vi "MAIN_static_friction.vi"() -> ()   [LabVIEW 2019]
uses:
  <vilib>/myRIO/Instrument Drivers/Onboard IO/AO/AO.lvlib
  <vilib>/myRIO/Instrument Drivers/Onboard IO/Encoder/Encoder.lvlib
  <vilib>/myRIO/Instrument Drivers/Onboard IO/AI/AI.lvlib
  <vilib>/addons/control/pid/NI_PID_pid.lvlib
  <vilib>/Analysis/3filter.llb/Filter Passband Type.ctl
  <vilib>/Analysis/NI_AALBase.lvlib
  <vilib>/ptbypt/NI_PtbyPt.lvlib
  <vilib>/platform/TimedLoop/XDataNode/XDataNode.xnode
  <vilib>/Platform/TimedLoop/XDataNode/timing_clust.ctl
  <vilib>/Platform/TimedLoop/XDataNode/XDNodeRunTimeDep.lvlib
  <vilib>/Platform/TimedLoop/XDataNode/wakeup.ctl
  <vilib>/Platform/TimedLoop/XDataNode/nitl_modes.ctl
  <vilib>/myRIO/Common/Instrument Driver Framework/myRIO v1.0/Encoder/typedefs/Encoder Signal Mode.ctl
  <vilib>/myRIO/Instrument Drivers/Onboard IO/AO/vis/myRIO AO Open.xnode
  <vilib>/myRIO/Instrument Drivers/Onboard IO/AO/typedefs/AO Reference.ctl
  <vilib>/myRIO/Common/Instrument Driver Framework/Utilities/typedefs/Analog Scaling Constants List.ctl
  <vilib>/myRIO/Common/Instrument Driver Framework/Utilities/typedefs/Analog Scaling Constants.ctl
  <vilib>/myRIO/Common/Instrument Driver Framework/myRIO v1.0/AO/typedefs/AO Channels List.ctl
  <vilib>/myRIO/Common/Instrument Driver Framework/myRIO v1.0/AO/typedefs/AO Channels Enum.ctl
  <vilib>/myRIO/Common/Instrument Driver Framework/Utilities/typedefs/myRIO Generic Hardware Reference.ctl
  <vilib>/myRIO/Common/Instrument Driver Framework/Utilities/typedefs/myRIO v1.0 Reference.ctl
  <vilib>/myRIO/Common/Instrument Driver Framework/Utilities/typedefs/Generic FPGA Reference.ctl
  <vilib>/myRIO/Common/Instrument Driver Framework/Utilities/typedefs/Hardware Version Enum.ctl
  <vilib>/userDefined/High Color/nirio_resource_hc.ctl
  <vilib>/myRIO/Common/Instrument Driver Framework/myRIO v1.0/AO/vis/myRIO v1.1 Open AO.vi
  <vilib>/myRIO/Instrument Drivers/Onboard IO/AI/vis/myRIO AI Open.xnode
  <vilib>/myRIO/Instrument Drivers/Onboard IO/AI/typedefs/AI Reference.ctl
  <vilib>/myRIO/Common/Instrument Driver Framework/myRIO v1.0/AI/typedefs/AI Channels List.ctl
  <vilib>/myRIO/Common/Instrument Driver Framework/myRIO v1.0/AI/typedefs/AI Channels Enum.ctl
  <vilib>/myRIO/Common/Instrument Driver Framework/myRIO v1.0/AI/vis/myRIO v1.1 Open AI.vi
  Shared VIs/TypeDef_TDMS_States.ctl
  TypeDef_Actions.ctl
  Shared VIs/ENPID/PID_Settings.ctl
  Shared VIs/ENPID/OutputRange.ctl
  Shared VIs/ENPID/VelocityEstimate.ctl
  Shared VIs/ENPID/DPartVariable.ctl
  Shared VIs/ENPID/NonLinearGain.ctl
  Shared VIs/ENPID/NonLinearGainParams.ctl
  Shared VIs/ENPID/Gains.ctl
  TypeDef_Current-Direction.ctl
panel:
  in  "Pos Difference \nThreshold [deg]":dbl=1.0 min=0.0 max=1.0 step=0.01 format="%#_13g"
  in  "Actions":T1
  in  "Current Direction":T2
  out "Position End [deg] Chart":dbl(graph)
  out "Position End [deg]":dbl
  out "Initial Position [deg]":dbl
  out "Velocity [deg/s] Chart":dbl(graph)
  in  "Stop saving data":bool
  in  "Save data?":bool
  in  "File Storage Name":string
  out "Final Current Setpoint":dbl
  out "Boolean: Apply Current":bool
  out "Boolean: Move":bool
  out "Position Difference [deg]":dbl
  in  "move":bool
  out "Profile Complete?":bool
  out "Velocity [deg/s]":dbl
  out "Current Setpoint [A]":dbl
  out "Position [deg] Chart":dbl(graph)
  out "Current [A] Chart":dbl(graph)
  out "Position [deg]":dbl
  in  "stop":bool
  out "Current [A]":dbl
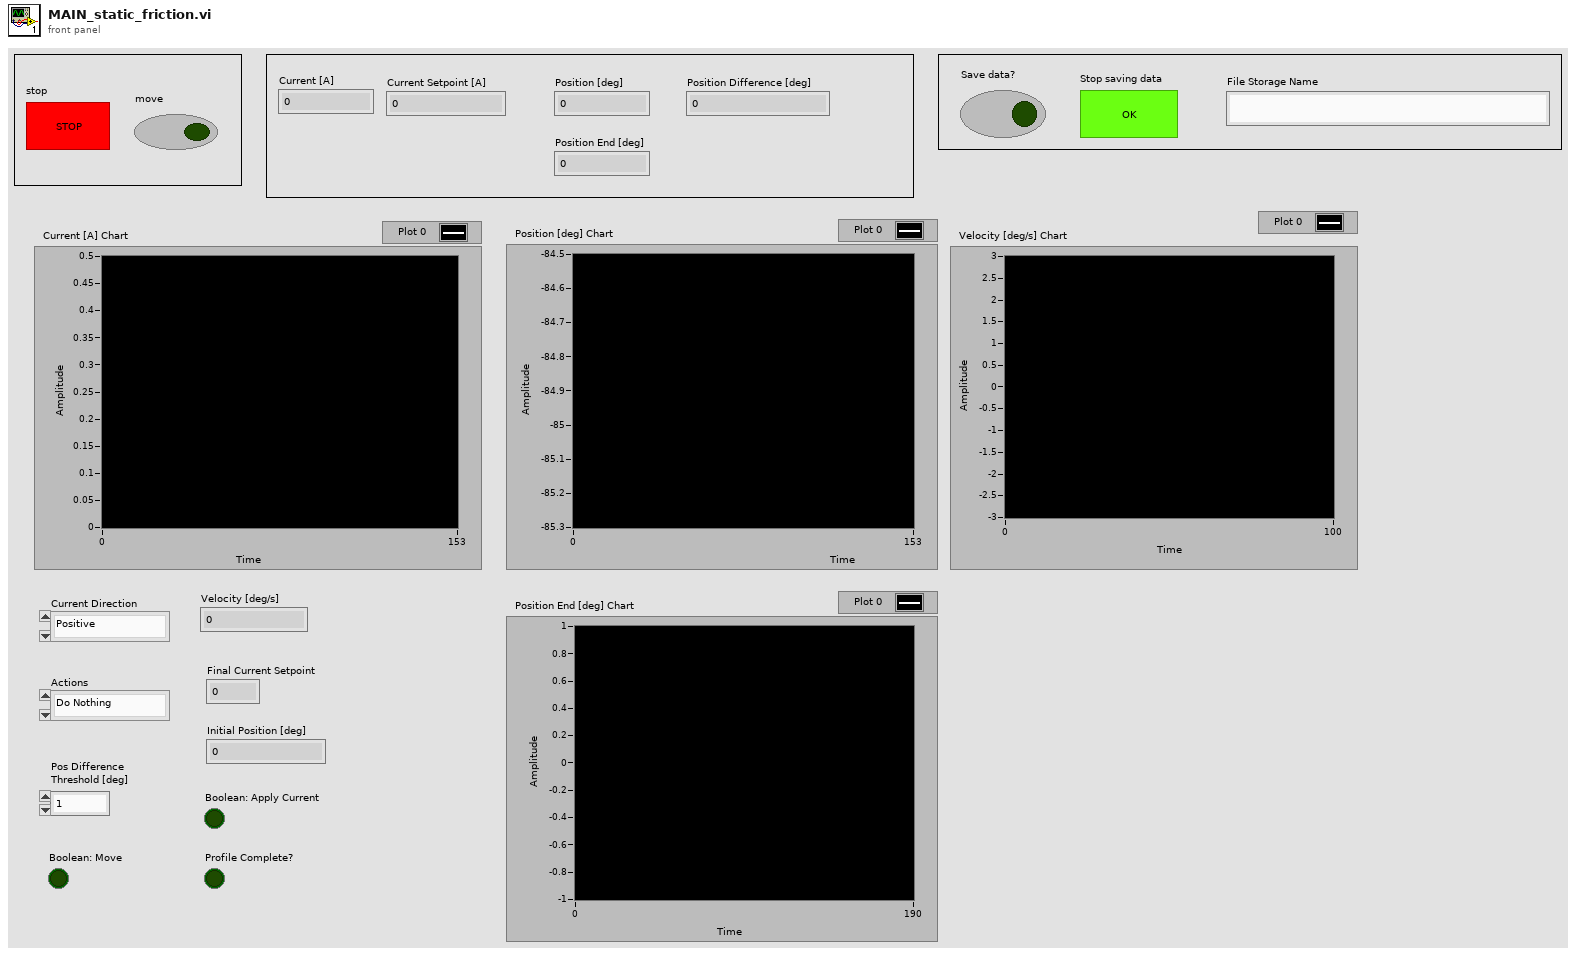
[diagram p1: front panel]
types:
  T1 = typedef "TypeDef_Actions.ctl" = enum16{"Do Nothing", "Move", "Wait", "Apply Current"}
  T2 = typedef "TypeDef_Current-Direction.ctl" = enum16{"Positive", "Negative"}
  T3 = typedef "nirio_resource_hc.ctl" = tag
  T4 = typedef "Hardware Version Enum.ctl" = enum16{"Unknown", "myRIO-1900", "myRIO-1950", "roboRIO", "NI ELVIS RIO CM", "ELVIS III"}
  T5 = typedef "TypeDef_TDMS_States.ctl" = enum16{"WaitingForCreate", "Create", "Buffering", "Flushing", "Write", "Close"}
  T6 = enum16{"open", "open or create", "create or replace", "create", "open (read-only)"}
  T7 = typedef "XDNodeRunTimeDep.lvlib/timing_clust.ctl" = cluster{"Expected End [f-1]":u64, "Actual End [f-1]":u64, "Finished Late? [f-1]":bool, "Expected End [i-1]":u64, "Actual End [i-1]":u64, "Finished Late? [i-1]":bool, "Expected Start [i]":u64, "Actual Start [i]":u64, "Expected Start [f]":u64, "Actual Start [f]":u64, "Source Name":string, "Structure Name":string, "Period":i64, "Deadline":i64, "Offset":i64, "Start":i64, "Priority":i32, "Timeout":i32, "Mode":T8, "Wakeup Reason":T9, "Error":errorcluster, "Source Type":string, "Secondary Source Type":string, "Global End Time":u64, "Global Start Time":u64, "Frame Duration":u64, "Iteration Duration":u64, "Assigned CPU":i32, "I/O Scan Engine Mode":u32}
  T8 = typedef "XDNodeRunTimeDep.lvlib/nitl_modes.ctl" = enum32{"No Change", "Process missed periods, maintain original phase", "Discard missed periods, maintain original phase", "Process missed periods, ignore original phase", "Discard missed periods, ignore original phase"}
  T9 = typedef "XDNodeRunTimeDep.lvlib/wakeup.ctl" = enum32{"Normal", "Aborted", "Asynchronous wakeup", "Timing source error", "Timed loop error", "Timeout"}
  T10 = typedef "NI_AALBase.lvlib/Filter Passband Type.ctl" = enum32{"Lowpass", "Highpass", "Bandpass", "Bandstop"}
  T11 = typedef "PID_Settings.ctl" = cluster{"Gains":T12, "Non-linear gain":T13, "D-Part variable":T15, "Velocity estimate dy/dt":T16, "Anti reset windup":bool, "I-Part error band":dbl, "Output range":T17}
  T12 = typedef "Gains.ctl" = cluster{"K(e)":dbl, "Kp":dbl, "Ki":dbl, "Kd":dbl}
  T13 = typedef "NonLinearGainParams.ctl" = cluster{"Non-linear gain P":T14, "Non-linear gain I":T14, "Non-linear gain D":T14}
  T14 = typedef "NonLinearGain.ctl" = enum16{"exponential", "quadratic", "off"}
  T15 = typedef "DPartVariable.ctl" = enum16{"error", "process variable"}
  T16 = typedef "VelocityEstimate.ctl" = enum16{"derivative", "external"}
  T17 = typedef "OutputRange.ctl" = cluster{"output high":dbl, "output low":dbl}
  T18 = typedef "Encoder Signal Mode.ctl" = enum16{"Quadrature phase signal", "Step and direction signal"}
  T19 = typedef "AO.lvlib/AO Reference.ctl" = cluster{"myRIO Reference":T20, "AO Channel List":T23, "AO Scaling Constant List":T25}
  T20 = typedef "myRIO Generic Hardware Reference.ctl" = cluster{"myRIO Model":T4, "myRIO Hardware Reference":T21}
  T21 = typedef "myRIO v1.0 Reference.ctl" = cluster{"Generic FPGA Reference":T22, "Allow multiple opens":bool}
  T22 = typedef "Generic FPGA Reference.ctl" = refnum<k20>
  T23 = typedef "AO Channels List.ctl" = T24[]
  T24 = typedef "AO Channels Enum.ctl" = enum16{"Not Connected", "AudioOut/Left", "AudioOut/Right", "C/AO0", "C/AO1", "A/AO0", "A/AO1", "B/AO0", "B/AO1"}
  T25 = typedef "Analog Scaling Constants List.ctl" = T26[]
  T26 = typedef "Analog Scaling Constants.ctl" = cluster{"LSB Weight (Volts)":dbl, "Offset (Volts)":dbl, "Signed?":bool}
  T27 = typedef "Encoder.lvlib/Encoder Reference.ctl" = cluster{"myRIO Reference":T20, "Encoder Channels Enum":T28}
  T28 = typedef "Encoder Channels Enum.ctl" = enum16{"Not Connected", "C/ENC0", "C/ENC1", "A/ENC", "A/ENC0", "A/ENC1", "A/ENC2", "A/ENC3", "A/ENC4", "A/ENC5", "A/ENC6", "A/ENC7", "A/ENC8", "A/ENC9", "B/ENC", "B/ENC0", "B/ENC1", "B/ENC2", "B/ENC3", "B/ENC4", "B/ENC5", "B/ENC6", "B/ENC7", "B/ENC8", "B/ENC9", "DIO/ENC0", "DIO/ENC1", "DIO/ENC2", "DIO/ENC3", "DIO/ENC4"}
  T29 = typedef "AI.lvlib/AI Reference.ctl" = cluster{"myRIO Reference":T20, "AI Channels List":T30, "AI Scaling Constants List":T25}
  T30 = typedef "AI Channels List.ctl" = T31[]
  T31 = typedef "AI Channels Enum.ctl" = enum16{"Not Connected", "AudioIn/Left", "AudioIn/Right", "C/AI0", "C/AI1", "A/AI0", "A/AI1", "A/AI2", "A/AI3", "A/AI4", "A/AI5", "A/AI6", "A/AI7", "B/AI0", "B/AI1", "B/AI2", "B/AI3", "B/AI4", "B/AI5", "B/AI6", "B/AI7", "AI/AI0", "AI/AI1", "AI/AI2", "AI/AI3", "A/AI0 (DIFF)", "A/AI1 (DIFF)", "A/AI2 (DIFF)", "A/AI3 (DIFF)", "B/AI0 (DIFF)", "B/AI1 (DIFF)", "B/AI2 (DIFF)", "B/AI3 (DIFF)"}
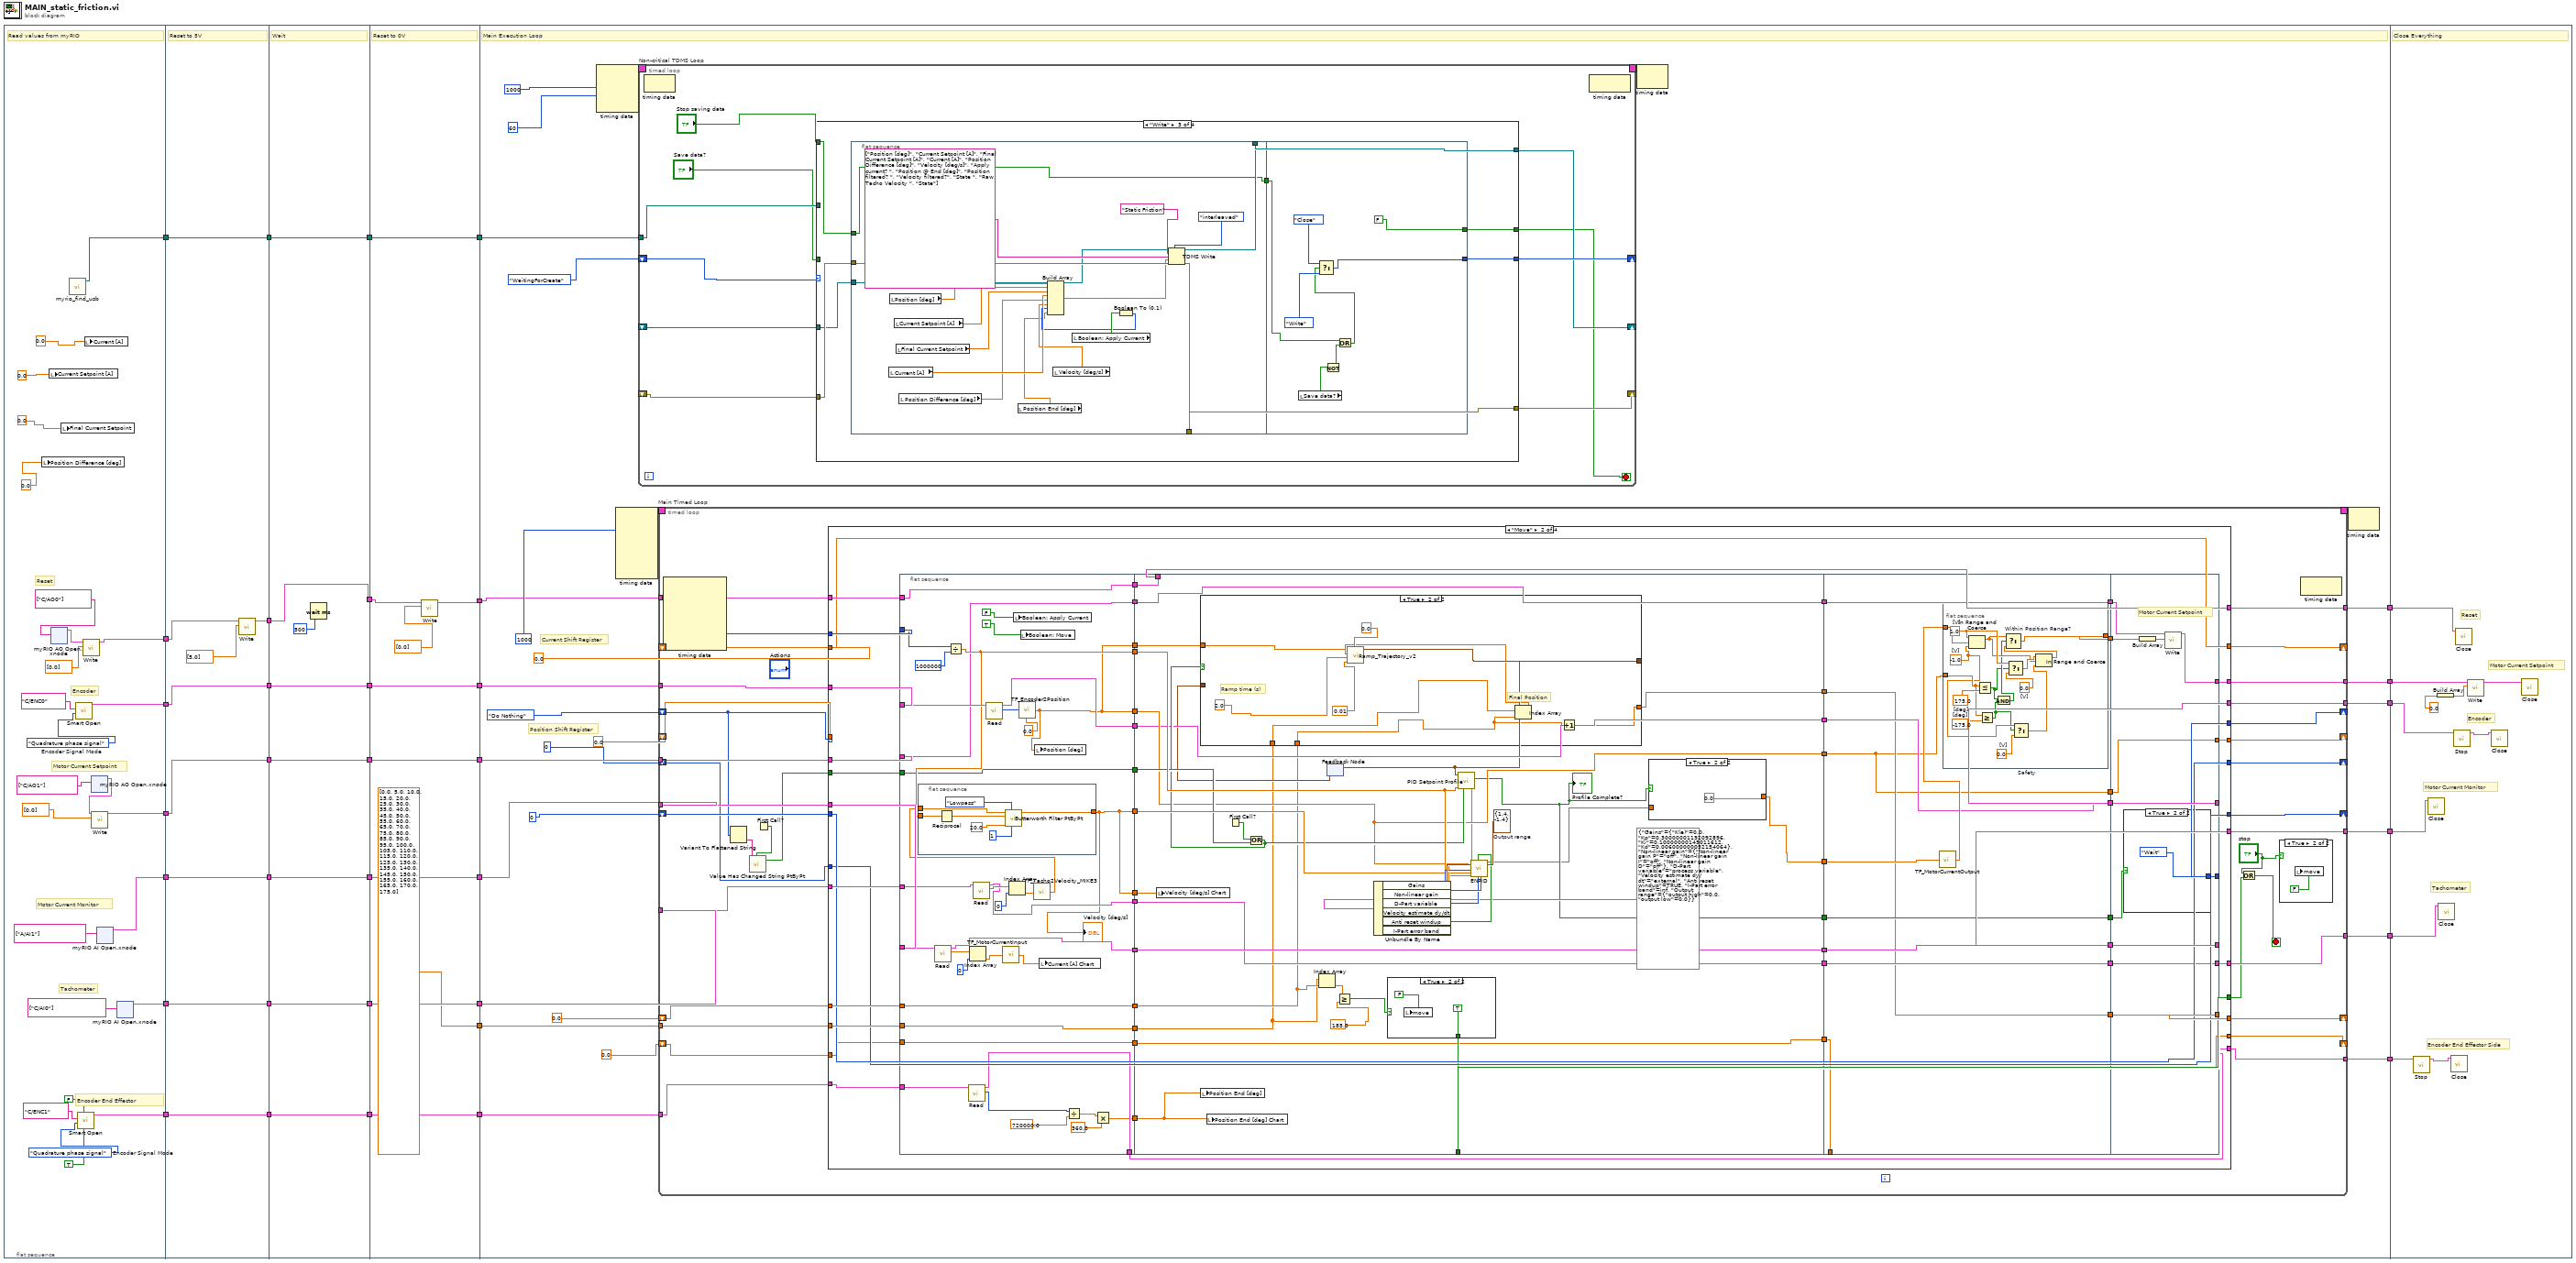
[diagram p0: block diagram]
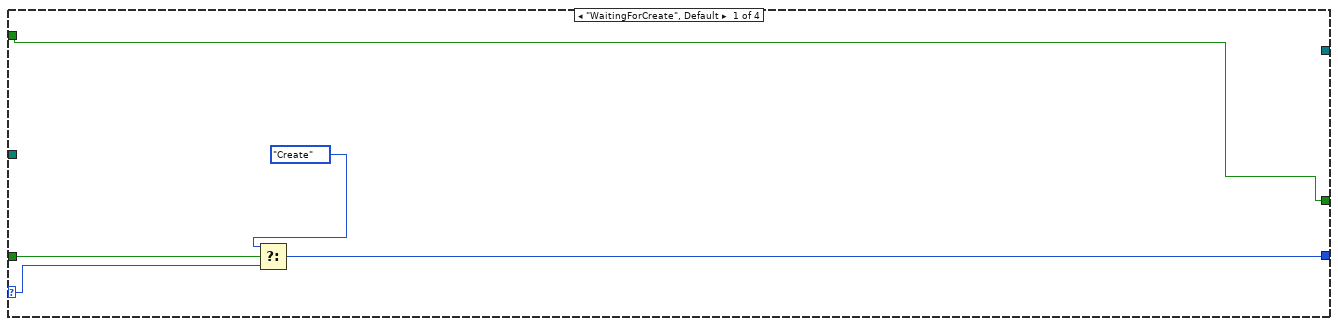
[diagram p2: hidden frame]
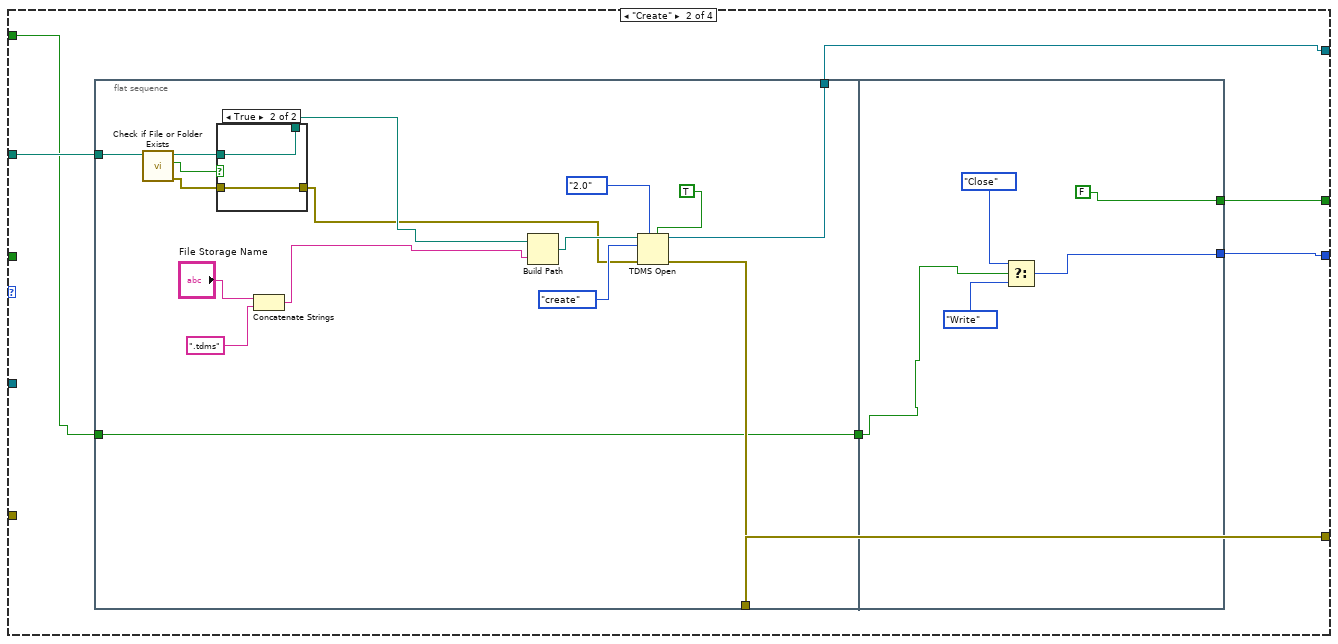
[diagram p3: hidden frame]
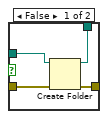
[diagram p4: hidden frame]
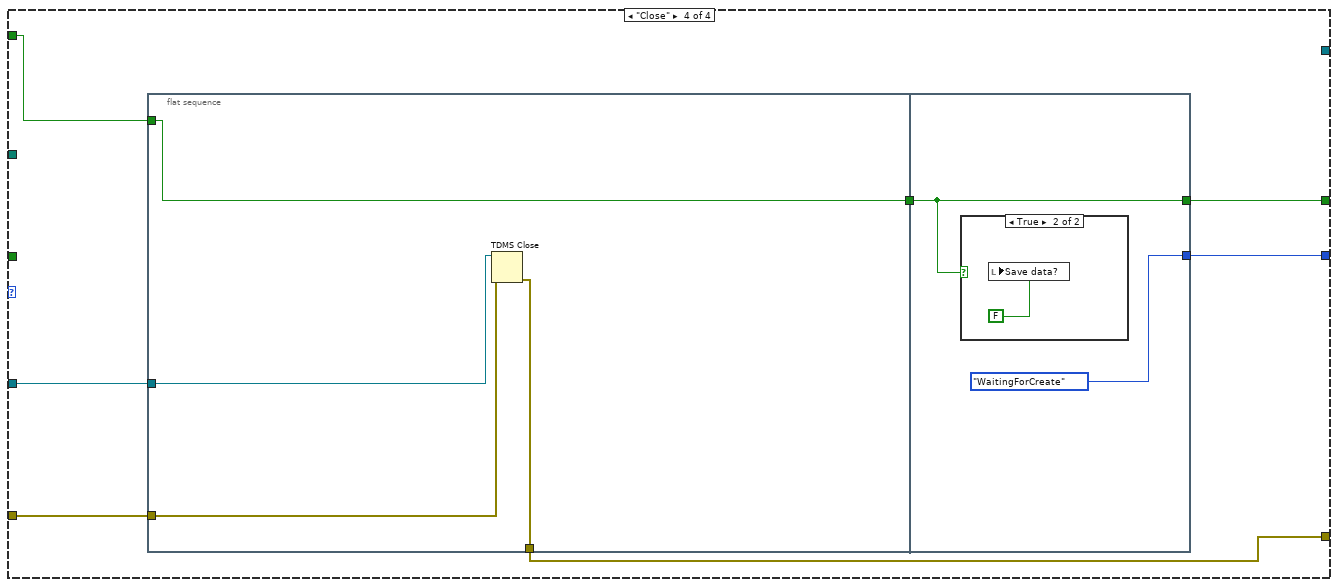
[diagram p5: hidden frame]
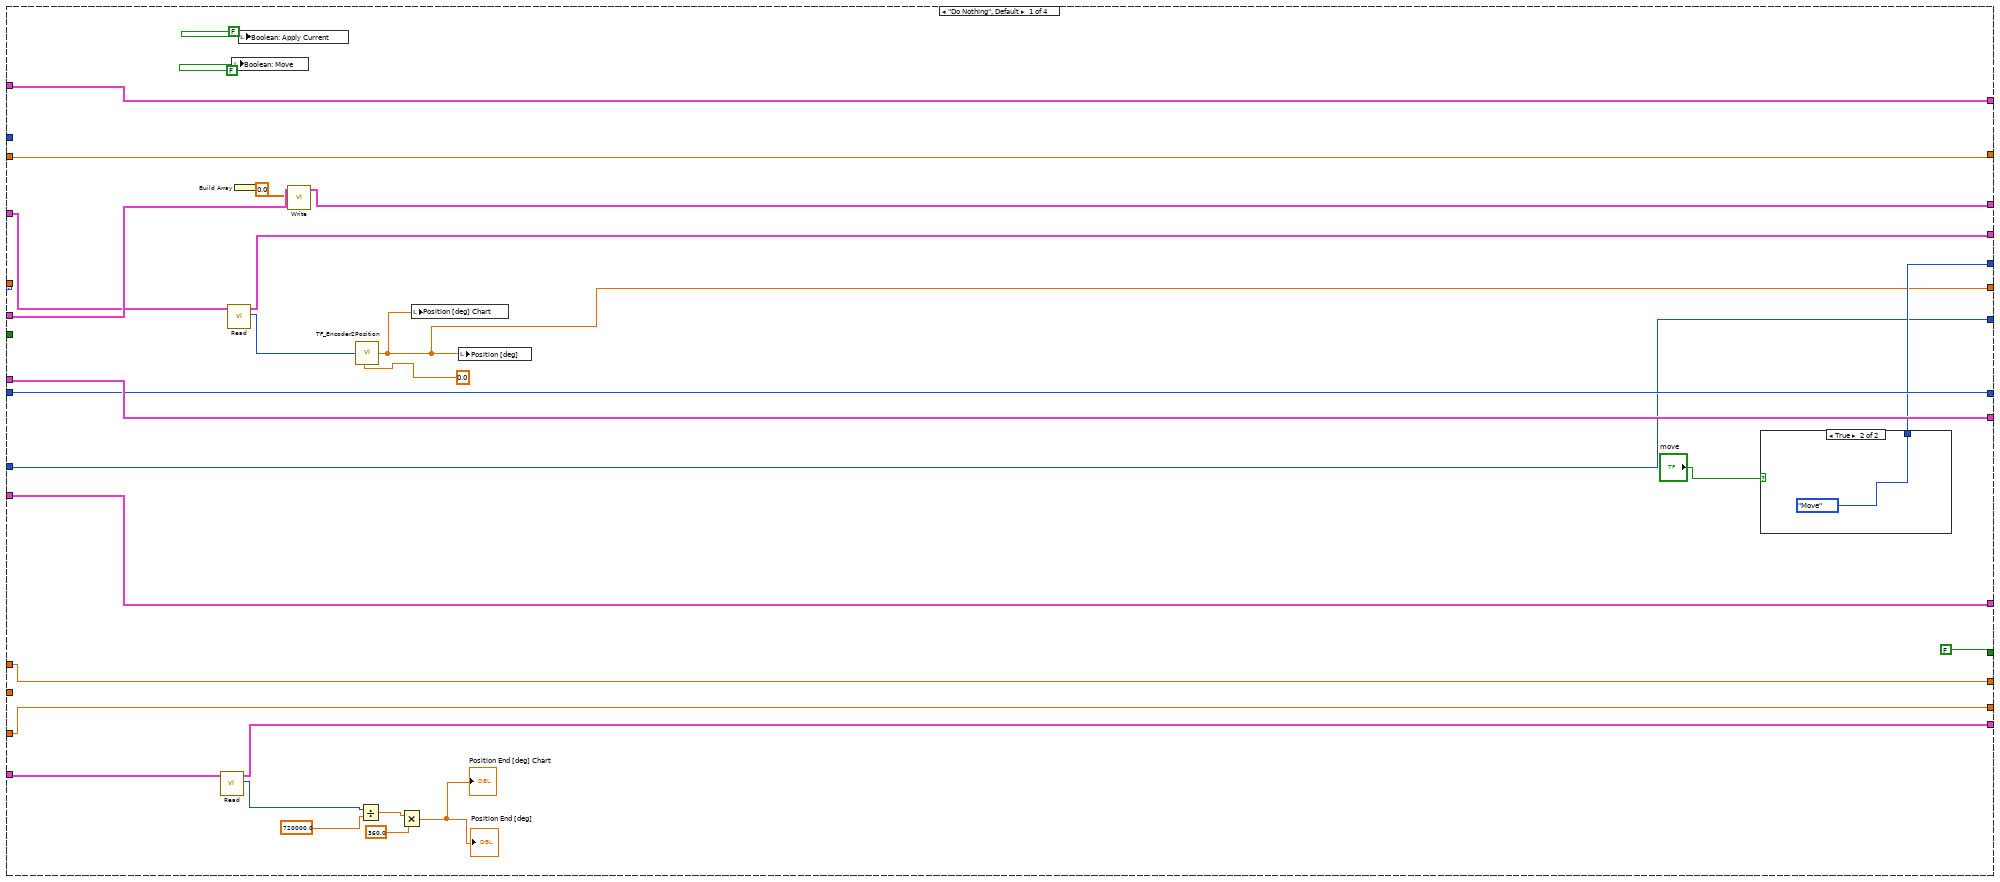
[diagram p8: hidden frame]
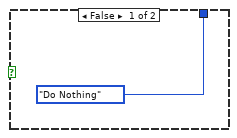
[diagram p9: hidden frame]
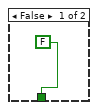
[diagram p10: hidden frame]
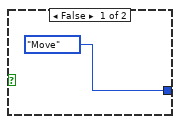
[diagram p13: hidden frame]
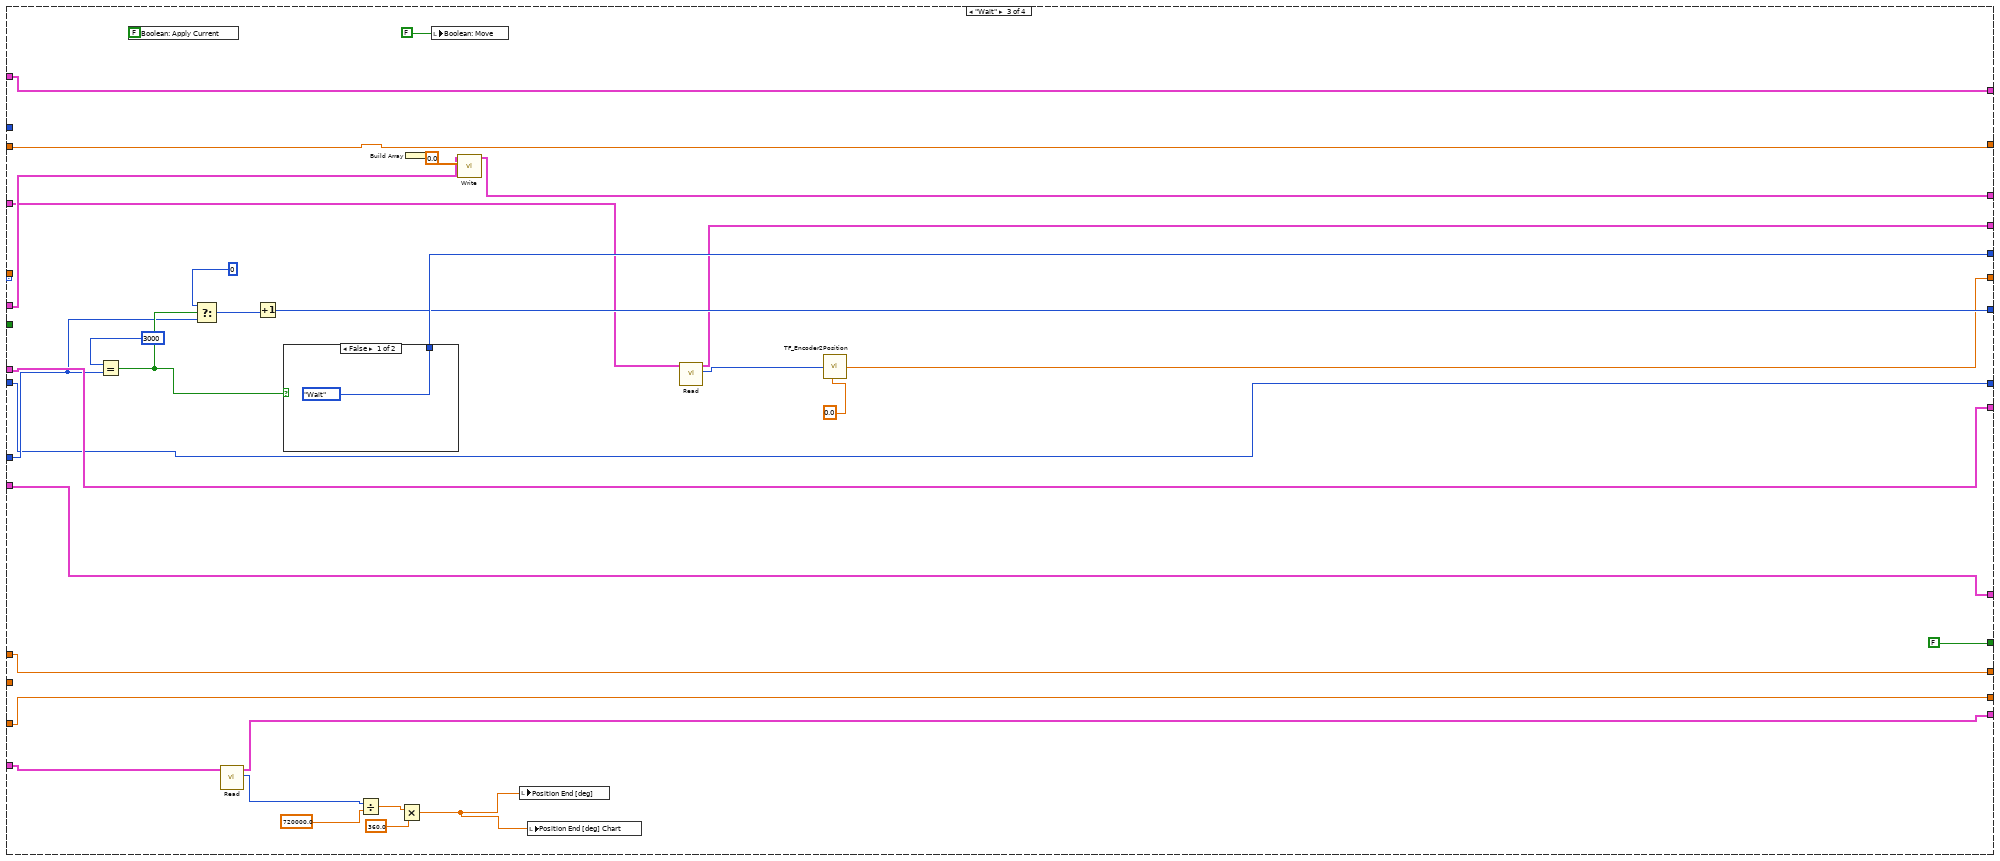
[diagram p14: hidden frame]
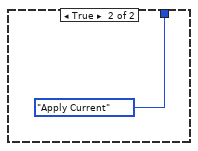
[diagram p15: hidden frame]
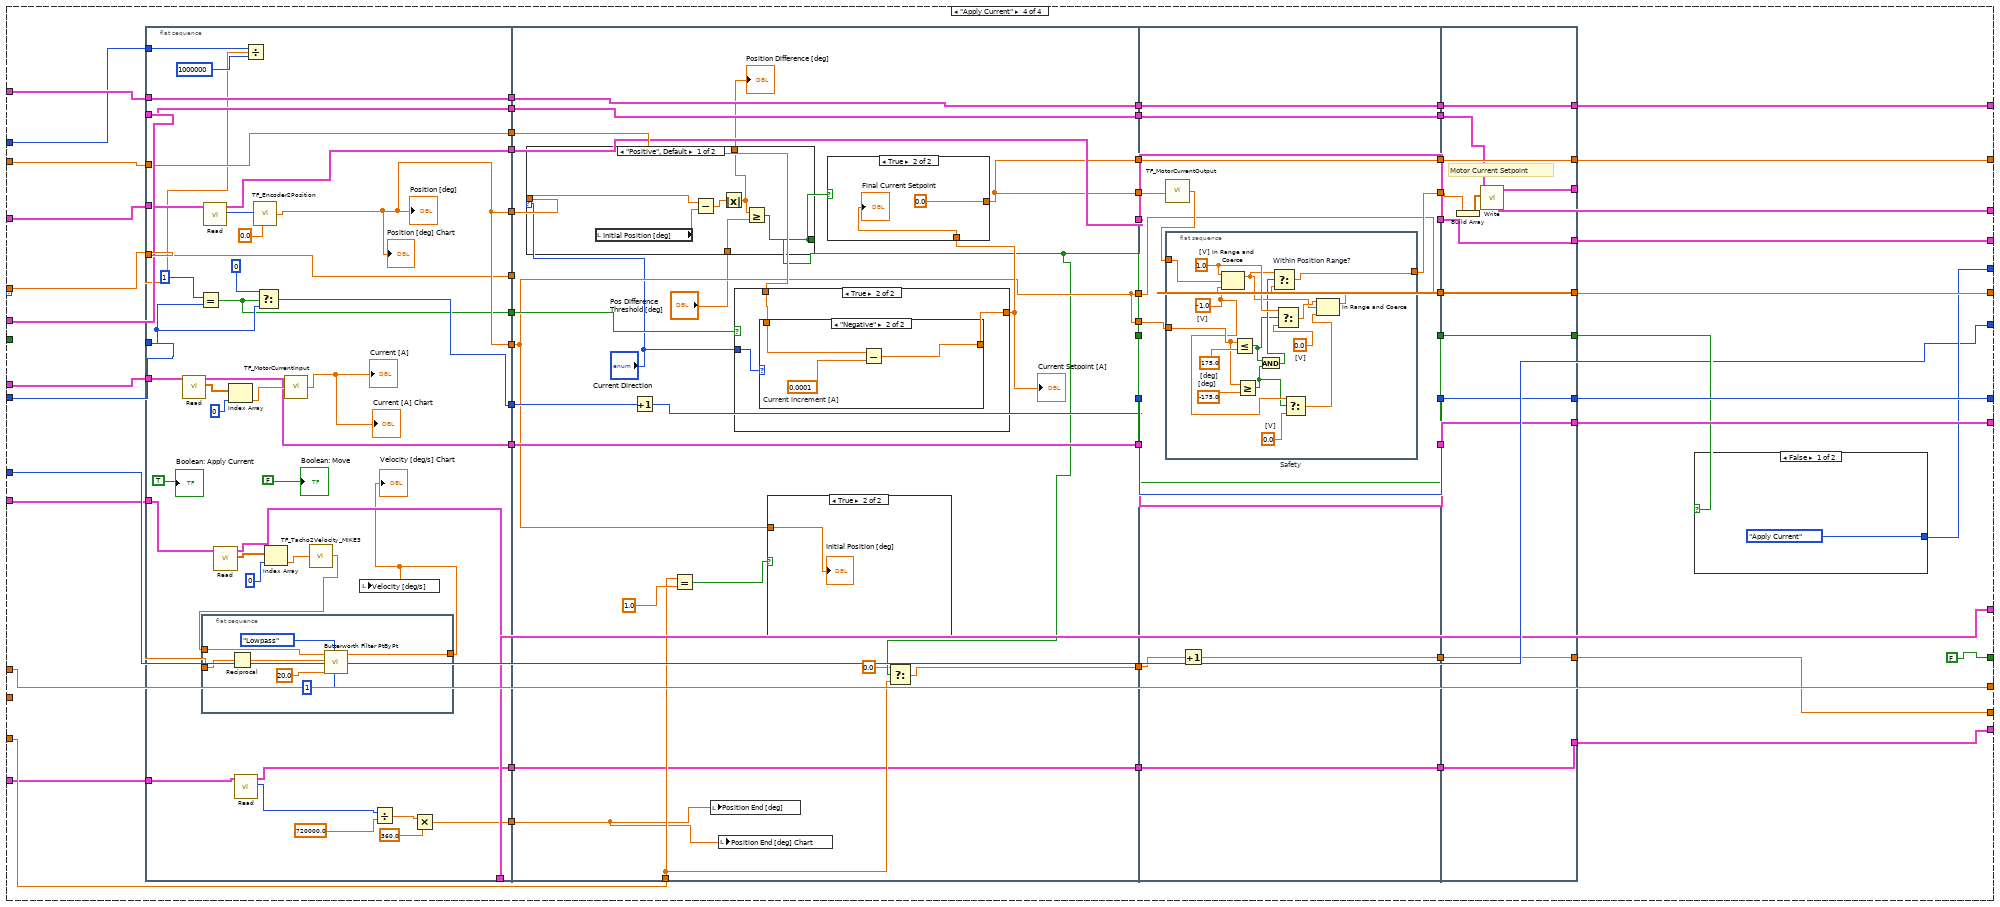
[diagram p16: hidden frame]
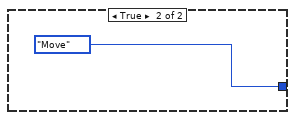
[diagram p17: hidden frame]
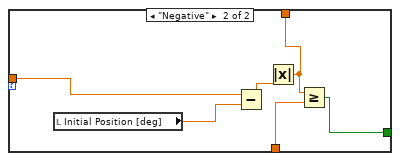
[diagram p19: hidden frame]
diagram:
  n1 = flat-sequence {
    tunnel: [w57] -> w35
    tunnel: [w54] -> w31
    tunnel: [w50] -> w30
    tunnel: [w48] -> w29
    tunnel: [w46] -> w12
    tunnel: [w45] -> w6
    tunnel: [w36] -> w2
    tunnel: w35 -> [w140]
    tunnel: [w139] -> w33
    tunnel: w31 -> [w138]
    tunnel: w30 -> [w137]
    tunnel: w29 -> [w136]
    tunnel: [w138] -> w26
    tunnel: [w137] -> w23
    tunnel: [w136] -> w20
    tunnel: [w135] -> w13
    tunnel: w12 -> [w135]
    tunnel: [w134] -> w7
    tunnel: w6 -> [w134]
    tunnel: [w133] -> w3
    tunnel: w2 -> [w133]
    tunnel: [w148] -> w34
    tunnel: w33 -> [w148]
    tunnel: [w147] -> w27
    tunnel: w26 -> [w147]
    tunnel: [w146] -> w24
    tunnel: w23 -> [w146]
    tunnel: [w145] -> w21
    tunnel: w20 -> [w145]
    tunnel: [w144] -> w14
    tunnel: w13 -> [w144]
    tunnel: [w143] -> w8
    tunnel: w7 -> [w143]
    tunnel: [w142] -> w4
    tunnel: w3 -> [w142]
    tunnel: w34 -> [w158]
    tunnel: [w157] -> w32
    tunnel: [w156] -> w28
    tunnel: w27 -> [w156]
    tunnel: [w155] -> w25
    tunnel: w24 -> [w155]
    tunnel: [w154] -> w22
    tunnel: w21 -> [w154]
    tunnel: [w153] -> w15
    tunnel: w14 -> [w153]
    tunnel: [dbl[] [0.0, 5.0, 10.0, 15.0, 20.0, 25.0, 30.0, 35.0, 40.0, 45.0, 50.0, 55.0, 60.0, 65.0, 70.0, 75.0, 80.0, 85.0, 90.0, 95.0, 100.0, 105.0, 110.0, 115.0, 120.0, 125.0, 130.0, 135.0, 140.0, 145.0, 150.0, 155.0, 160.0, 165.0, 170.0, 175.0]] -> w10
    tunnel: [w151] -> w9
    tunnel: w8 -> [w151]
    tunnel: [w150] -> w5
    tunnel: w4 -> [w150]
    tunnel: w32 -> [w181]
    tunnel: w28 -> [w185]
    tunnel: w25 -> [w184]
    tunnel: w22 -> [w175]
    tunnel: [w180] -> w19
    tunnel: [w179] -> w18
    tunnel: [w178] -> w17
    tunnel: [w177] -> w16
    tunnel: w15 -> [w176]
    tunnel: [w174] -> w11
    tunnel: w10 -> [w173]
    tunnel: w9 -> [w166]
    tunnel: w5 -> [w162]
    tunnel: [w161] -> w1
    tunnel: w19 -> [w805]
    tunnel: w18 -> [w800]
    tunnel: w17 -> [w799]
    tunnel: w16 -> [w798]
    tunnel: w11 -> [w797]
    tunnel: w1 -> [w795]
    frame #0 {
      w39 = Encoder_Signal_Mode."Quadrature phase signal"  # Encoder Signal Mode
      w55 = Encoder_Signal_Mode."Quadrature phase signal"  # Encoder Signal Mode
      # "Encoder End Effector"
      # "Tachometer"
      # "Motor Current Monitor"
      # "Motor Current Setpoint"
      # "Encoder"
      # "Reset"
      # "Read values from myRIO"
      n2 = local write "Position Difference [deg]"(0.0) -> ()
      n3 = local write "Current Setpoint [A]"(0.0) -> ()
      n4 = xnode "myRIO AO Open.xnode"("Channel Names"=tag[] ["C/AO0"]) -> ("AO Ref Out"=w59:T19)  [unwired: 2 in, 1 out]
      n5 = local write "Final Current Setpoint"(0.0) -> ()
      n6 = call "myrio_find_usb.vi"() -> ("Largest USB Partition Path"=w45:path)  [unwired: 9 in, 2 out]
      n7 = call <vilib>:"Smart Open.vi"("Encoder Signal Mode"=w55, "Channel Name"=tag "C/ENC0") -> ("Encoder Ref Out"=w54:T27)  [unwired: 8 in, 1 out]
      n8 = call <vilib>:"Smart Open.vi"("Start Counter"=TRUE, "Allow multiple opens?"=FALSE, "Encoder Signal Mode"=w39, "Channel Name"=tag "C/ENC1") -> ("Encoder Ref Out"=w36:T27)  [unwired: 6 in, 1 out]
      n9 = call <vilib>:"Write.vi"("Values"=dbl[] [0.0], "AO Ref In"=w59) -> ("AO Ref Out"=w57:T19)  [unwired: 7 in, 1 out]
      n10 = local write "Current [A]"(0.0) -> ()
      n11 = xnode "myRIO AO Open.xnode"("Channel Names"=tag[] ["C/AO1"]) -> ("AO Ref Out"=w52:T19)  [unwired: 2 in, 1 out]
      n12 = call <vilib>:"Write.vi"("Values"=dbl[] [0.0], "AO Ref In"=w52) -> ("AO Ref Out"=w50:T19)  [unwired: 7 in, 1 out]
      n13 = xnode "myRIO AI Open.xnode"("Channel Names"=tag[] ["A/AI1"]) -> ("AI Ref Out"=w48:T29)  [unwired: 2 in, 1 out]
      n14 = xnode "myRIO AI Open.xnode"("Channel Names"=tag[] ["C/AI0"]) -> ("AI Ref Out"=w46:T29)  [unwired: 2 in, 1 out]
    }
    frame #1 {
      # "Reset to 5V"
      n15 = call <vilib>:"Write.vi"("Values"=dbl[] [5.0], "AO Ref In"=w140) -> ("AO Ref Out"=w139:T19)  [unwired: 7 in, 1 out]
    }
    frame #2 {
      # "Wait"
      n16 = Wait (ms)(milliseconds to wait=500) -> ()  [unwired: 1 out]
    }
    frame #3 {
      # "Reset to 0V"
      n17 = call <vilib>:"Write.vi"("Values"=dbl[] [0.0], "AO Ref In"=w158) -> ("AO Ref Out"=w157:T19)  [unwired: 7 in, 1 out]
    }
    frame #4 {
      # "Position Shift Register"
      # "Current Shift Register"
      # "Main Execution Loop"
      n18 = node-c288(1000, 60) -> (w170:T7)  [unwired: 2 in]
      n19 = node-c288(1000) -> (w188:T7)  [unwired: 6 in]
      n20 = timed-loop "Non-critical TDMS Loop" {
        timing: w170 -> [_]
        timing-out: [_] -> w169
        tunnel: w166 -> [w196]
        shift-right: [w198] -> _
        shift-left: TypeDef_TDMS_States."WaitingForCreate" ("TDMS States") -> [w197]
        shift-right: [w195] -> _
        shift-left: _ -> [w192]
        shift-right: [w194] -> _
        shift-left: _ -> [w193]
        stop <- w191 stop-if-true
        n21 = node-c288() -> ()  [unwired: 1 in, 1 out]
        n22 = case shown="\"Write\"" w197 {
          selector: w197 -> [w201 _ _ _]
          tunnel: "Save data?" -> [w202 _ _ _]
          tunnel: [w200 w207 w242 w275] -> w198
          tunnel: w196 -> [_ w210 _ _]
          tunnel: [_ w208 w243 _] -> w195
          tunnel: [_ w209 w245 w276] -> w194
          tunnel: w193 -> [_ _ w244 w277]
          tunnel: w192 -> [_ _ w240 w278]
          tunnel: [w199 w206 w241 w274] -> w191
          tunnel: "Stop saving data" -> [w199 w204 w238 w273]
          frame "WaitingForCreate", Default {
            n23 = Select(t=TypeDef_TDMS_States."Create" ("TDMS States"), s=w202, f=w201) -> (s? t:f=w200:T5)
          }
          frame "Create" {
            n24 = flat-sequence {
              tunnel: w210 -> [w226]
              tunnel: [w214] -> w209
              tunnel: [w213] -> w208
              tunnel: [w211] -> w205
              tunnel: w204 -> [w211]
              tunnel: [w235] -> w207
              tunnel: [FALSE] -> w206
              tunnel: w205 -> [w233]
              frame #0 {
                n25 = call <vilib>:"Check if File or Folder Exists.vi"("path"=w226) -> ("error out"=w224:errorcluster, "file or folder exists?"=w212:bool, "dup path"=w225:path)  [unwired: 8 in]
                n26 = case shown="True" w212 {
                  tunnel: w225 -> [w230 w231]
                  tunnel: [w229 w232] -> w215
                  tunnel: w224 -> [w228 w232]
                  tunnel: [w227 w231] -> w216
                  frame False {
                    n27 = Create Folder(path (use dialog)=w230, error in=w228) -> (created path=w227:path, error out=w229:errorcluster)  [unwired: 1 in, 1 out]
                  }
                  frame True {
                  }
                }
                n28 = Concatenate Strings("File Storage Name", ".tdms") -> (w217:string)
                n29 = Build Path(base path=w216, name or relative path=w217) -> (appended path=w221:path)
                n30 = TDMS Open(5:TRUE, 7:enum16{"1.0", "2.0"}."2.0" ("file format version (2.0)"), 8:w215, 10:T6."create" ("operation (0:open)"), 11:w221) -> (0:w214:errorcluster, 3:w213:refnum<k34>)  [unwired: 2 in]
              }
              frame #1 {
                n31 = Select(t=TypeDef_TDMS_States."Close" ("TDMS States"), s=w233, f=TypeDef_TDMS_States."Write" ("TDMS States")) -> (s? t:f=w235:T5)
              }
            }
          }
          frame "Write" {
            n32 = flat-sequence {
              tunnel: [w261] -> w245
              tunnel: w244 -> [w260]
              tunnel: [w252] -> w243
              tunnel: w240 -> [w251]
              tunnel: w238 -> [w250]
              tunnel: [w250] -> w239
              tunnel: [w269] -> w242
              tunnel: [FALSE] -> w241
              tunnel: w239 -> [w265]
              frame #0 {
                n33 = local read "Current [A]"() -> (w255:dbl)
                n34 = local read "Position [deg]"() -> (w258:dbl)
                n35 = local read "Current Setpoint [A]"() -> (w257:dbl)
                n36 = local read "Final Current Setpoint"() -> (w256:dbl)
                n37 = local read "Position Difference [deg]"() -> (w254:dbl)
                n38 = local read "Position End [deg]"() -> (w246:dbl)
                n39 = local read "Velocity [deg/s]"() -> (w249:dbl)
                n40 = local read "Boolean: Apply Current"() -> (w248:bool)
                n41 = Boolean To (0,1)(Boolean=w248) -> (0, 1=w247:i16)
                n42 = Build Array(w258, w257, w256, w255, w254, w249, w247, w246) -> (w253:dbl[])
                n43 = TDMS Write(0:w251, 1:enum16{"decimated", "interleaved"}."interleaved" ("data layout (0:decimated)"), 5:"Static Friction" ("group name in (Untitled)"), 7:string[] ["Position [deg]", "Current Setpoint [A]", "Final Current Setpoint [A]", "Current [A]", "Position Difference [deg]", "Velocity [deg/s]", "Apply current? ", "Position @ End [deg]", "Position filtered? ", "Velocity filtered?", "State ", "Raw Tacho Velocity ", "State"], 9:w253, 11:w260) -> (4:w252:refnum<k34>, 15:w261:errorcluster)  [unwired: 2 out]
              }
              frame #1 {
                n44 = local read "Save data?"() -> (w267:bool)
                n45 = Not(x=w267) -> (.not. x?=w266:bool)
                n46 = Or(x=w265, y=w266) -> (x .or. y?=w264:bool)
                n47 = Select(t=TypeDef_TDMS_States."Close" ("TDMS States"), s=w264, f=TypeDef_TDMS_States."Write" ("TDMS States")) -> (s? t:f=w269:T5)
              }
            }
          }
          frame "Close" {
            n48 = flat-sequence {
              tunnel: w278 -> [w282]
              tunnel: w277 -> [w281]
              tunnel: [w280] -> w276
              tunnel: w273 -> [w279]
              tunnel: [w279] -> w272
              tunnel: [TypeDef_TDMS_States."WaitingForCreate" ("TDMS States")] -> w275
              tunnel: [w283] -> w274
              tunnel: w272 -> [w283]
              frame #0 {
                n49 = TDMS Close(8:w281, 11:w282) -> (0:w280:errorcluster)  [unwired: 1 out]
              }
              frame #1 {
                n50 = case shown="True" w283 {
                  frame False {
                  }
                  frame True {
                    n51 = local write "Save data?"(FALSE) -> ()
                  }
                }
              }
            }
          }
        }
        n52 = node-c288() -> ()  [unwired: 1 in, 1 out]
      }
      n53 = timed-loop "Main Timed Loop" {
        timing: w188 -> [_]
        timing-out: [_] -> w187
        tunnel: w185 -> [w325]
        tunnel: w184 -> [w318]
        tunnel: w175 -> [w326]
        shift-right: [w324] -> _
        shift-left: 0.0 -> [w323]
        shift-right: [w322] -> _
        shift-left: 0 -> [w321]
        shift-right: [w320] -> _
        shift-left: 0.0 ("Position [deg]") -> [w319]
        tunnel: w181 -> [w317]
        tunnel: [w316] -> w180
        tunnel: [w315] -> w179
        tunnel: [w311] -> w178
        tunnel: [w314] -> w177
        tunnel: w176 -> [w312]
        tunnel: [w310] -> w174
        shift-right: [w307] -> _
        shift-left: TypeDef_Actions."Do Nothing" ("Actions") -> [w306]
        tunnel: w173 -> [w304]
        shift-right: [w303] -> _
        shift-left: 0.0 -> [w302]
        shift-right: [w299] -> _
        shift-left: 0 -> [w298]
        shift-right: [w296] -> _
        shift-left: 0.0 -> [w295]
        tunnel: w162 -> [w294]
        tunnel: [w293] -> w161
        stop <- w301 stop-if-true
        n54 = node-c288() -> (w313:i64)  [unwired: 1 in, 7 out]
        n55 = Variant To Flattened String(Variant=w306) -> (data string=w309:string)  [unwired: 1 out]
        n56 = First Call?() -> (First Call?: T/F=w308:bool)
        n57 = call "Value Has Changed String PtByPt.vi"("input data point"=w309, "initialize"=w308) -> ("has changed"=w305:bool)  [unwired: 1 out]
        n58 = case shown="\"Move\"" w306 {
          tunnel: w326 -> [w354 w412 w572 w617]
          tunnel: w325 -> [w343 w414 w562 w616]
          tunnel: [w355 w371 w573 w615] -> w324
          tunnel: w323 -> [w355 w371 w573 w614]
          tunnel: [w353 w369 w567 w613] -> w322
          tunnel: w321 -> [w353 w370 w567 w612]
          tunnel: [w336 w368 w559 w611] -> w320
          tunnel: w319 -> [_ _ _ w610]
          tunnel: w318 -> [w350 w411 w578 w609]
          tunnel: w317 -> [w356 w409 w581 w608]
          tunnel: [w356 w408 w581 w607] -> w316
          tunnel: [w348 w410 w577 w606] -> w315
          tunnel: [w342 w407 w563 w605] -> w311
          tunnel: [w354 w406 w572 w604] -> w314
          tunnel: w313 -> [_ w415 _ w596]
          tunnel: w312 -> [w352 w413 w571 w598]
          tunnel: [w352 w405 w571 w597] -> w310
          tunnel: [w346 w381 w579 w602] -> w307
          tunnel: w305 -> [_ w382 _ _]
          tunnel: w304 -> [_ w379 _ _]
          tunnel: [w344 w375 w569 w600] -> w303
          tunnel: w302 -> [w344 w374 w569 w600]
          tunnel: [FALSE w373 FALSE FALSE] -> w300
          tunnel: w298 -> [w339 w369 w568 w599]
          tunnel: [w339 w370 w566 w599] -> w299
          tunnel: w295 -> [w335 w364 w558 w595]
          tunnel: [w335 w362 w558 w592] -> w296
          tunnel: w294 -> [w330 w361 w553 w591]
          tunnel: [w328 w360 w551 w590] -> w293
          frame "Do Nothing", Default {
            n59 = call <vilib>:"Read.vi"("Encoder Ref In"=w330) -> ("Counter Value"=w331:i32, "Encoder Ref Out"=w328:T27)  [unwired: 6 in, 3 out]
            n60 = call <vilib>:"Read.vi"("Encoder Ref In"=w343) -> ("Counter Value"=w341:i32, "Encoder Ref Out"=w342:T27)  [unwired: 6 in, 3 out]
            n61 = local write "Boolean: Move"(FALSE) -> ()
            n62 = Build Array(0.0) -> (w349:dbl[])
            n63 = local write "Boolean: Apply Current"(FALSE) -> ()
            n64 = call <vilib>:"Write.vi"("Values"=w349, "AO Ref In"=w350) -> ("AO Ref Out"=w348:T19)  [unwired: 7 in, 1 out]
            n65 = call "TF_Encoder2Position.vi"("Counter Value"=w341, "Offset"=0.0) -> ("Position [deg]"=w336:dbl)  [unwired: 3 in]
            n66 = Divide(x=w331, y=720000.0) -> (x/y=w333:dbl)
            n67 = Multiply(x=w333, y=360.0) -> (x*y=→"Position End [deg]" →"Position End [deg] Chart":dbl)
            n68 = local write "Position [deg] Chart"(w336) -> ()
            n69 = local write "Position [deg]"(w336) -> ()
            n70 = case shown="True" "move" {
              tunnel: [TypeDef_Actions."Do Nothing" ("Actions") TypeDef_Actions."Move" ("Actions")] -> w346
              frame False {
              }
              frame True {
              }
            }
          }
          frame "Move" {
            n71 = flat-sequence {
              tunnel: w415 -> [w444]
              tunnel: w414 -> [w450]
              tunnel: [w429] -> w404
              tunnel: w413 -> [w447]
              tunnel: [w443] -> w403
              tunnel: [w426] -> w402
              tunnel: w412 -> [w438]
              tunnel: w411 -> [w437]
              tunnel: [w437] -> w401
              tunnel: w382 -> [w436]
              tunnel: [w436] -> w400
              tunnel: [w435] -> w399
              tunnel: w409 -> [w435]
              tunnel: [w434] -> w398
              tunnel: [w433] -> w397
              tunnel: [w432] -> w396
              tunnel: [w431] -> w380
              tunnel: w374 -> [w431]
              tunnel: w379 -> [w430]
              tunnel: [w430] -> w378
              tunnel: [w429] -> w372
              tunnel: [w426] -> w366
              tunnel: [w425] -> w365
              tunnel: w364 -> [w425]
              tunnel: w361 -> [w420]
              tunnel: [w419] -> w360
              tunnel: [w418] -> w359
              tunnel: w404 -> [w481]
              tunnel: w403 -> [w485]
              tunnel: w402 -> [w486]
              tunnel: w401 -> [w479]
              tunnel: [w470] -> w395
              tunnel: w400 -> [w483]
              tunnel: [w481] -> w394
              tunnel: w399 -> [w480]
              tunnel: [w480] -> w408
              tunnel: [w479] -> w393
              tunnel: [w478] -> w392
              tunnel: w398 -> [w478]
              tunnel: w397 -> [w477]
              tunnel: [w477] -> w391
              tunnel: w396 -> [w476]
              tunnel: [w476] -> w390
              tunnel: [w472] -> w389
              tunnel: w380 -> [w465]
              tunnel: w378 -> [w464]
              tunnel: [w469] -> w377
              tunnel: [w467] -> w373
              tunnel: w372 -> [w466]
              tunnel: w366 -> [w461]
              tunnel: w365 -> [w460]
              tunnel: [w460] -> w363
              tunnel: w359 -> [w459]
              tunnel: w395 -> [w521]
              tunnel: w394 -> [w512]
              tunnel: [w519] -> w388
              tunnel: [w518] -> w387
              tunnel: w393 -> [w518]
              tunnel: w392 -> [w517]
              tunnel: [w517] -> w386
              tunnel: w391 -> [w516]
              tunnel: [w516] -> w385
              tunnel: [w515] -> w384
              tunnel: w390 -> [w515]
              tunnel: [w514] -> w383
              tunnel: w389 -> [w514]
              tunnel: w377 -> [w513]
              tunnel: [w513] -> w376
              tunnel: [w512] -> w367
              tunnel: w363 -> [w511]
              tunnel: [w511] -> w362
              tunnel: w388 -> [w548]
              tunnel: [w546] -> w410
              tunnel: w387 -> [w545]
              tunnel: w386 -> [w544]
              tunnel: [w544] -> w407
              tunnel: [w543] -> w406
              tunnel: w385 -> [w543]
              tunnel: [w542] -> w405
              tunnel: w384 -> [w542]
              tunnel: w383 -> [w541]
              tunnel: [w540] -> w381
              tunnel: [w539] -> w375
              tunnel: w376 -> [w539]
              tunnel: [w538] -> w368
              tunnel: w367 -> [w538]
              frame #0 {
                n72 = flat-sequence {
                  tunnel: w417 -> [w458]
                  tunnel: w443 -> [w456]
                  tunnel: [w453] -> w426
                  frame #0 {
                    n73 = Reciprocal(x=w456) -> (1/x=w457:dbl)
                    n74 = call <vilib>:"Butterworth Filter PtByPt.vi"("order"=1, "filter type"=Filter_Passband_Type."Lowpass", "low cutoff freq: fl"=20.0, "sampling freq: fs"=w457, "x"=w458) -> ("Filtered x"=w453:dbl)  [unwired: 4 in, 1 out]
                  }
                }
                n75 = call <vilib>:"Read.vi"("AI Ref In"=w438) -> ("Values"=w441:dbl[], "AI Ref Out"=w433:T29)  [unwired: 8 in, 1 out]
                n76 = Divide(x=w444, y=1000000) -> (x/y=w443:dbl)
                n77 = call <vilib>:"Read.vi"("Encoder Ref In"=w420) -> ("Counter Value"=w421:i32, "Encoder Ref Out"=w419:T27)  [unwired: 6 in, 3 out]
                n78 = Index Array(array=w441, index=0) -> (element=w440:dbl)
                n79 = call <vilib>:"Read.vi"("AI Ref In"=w447) -> ("Values"=w446:dbl[], "AI Ref Out"=w432:T29)  [unwired: 8 in, 1 out]
                n80 = call <vilib>:"Read.vi"("Encoder Ref In"=w450) -> ("Counter Value"=w449:i32, "Encoder Ref Out"=w434:T27)  [unwired: 6 in, 3 out]
                n81 = call "TF_MotorCurrentInput.vi"("Motor Current Monitor Value [V]"=w440) -> ("Current [A]"=w439:dbl)
                n82 = Index Array(array=w446, index=0) -> (element=w416:dbl)
                n83 = local write "Boolean: Apply Current"(FALSE) -> ()
                n84 = call "TF_Encoder2Position.vi"("Counter Value"=w449, "Offset"=0.0) -> ("Position [deg]"=w429:dbl)  [unwired: 3 in]
                n85 = local write "Boolean: Move"(TRUE) -> ()
                n86 = call "TF_Tacho2Velocity_MIKE3.vi"("Motor Velocity Tacho Value [V]"=w416) -> ("Motor Velocity Tacho [deg/s]"=w417:dbl)  [unwired: 4 in]
                n87 = local write "Position [deg]"(w429) -> ()
                n88 = local write "Current [A] Chart"(w439) -> ()
                n89 = Divide(x=w421, y=720000.0) -> (x/y=w423:dbl)
                n90 = Multiply(x=w423, y=360.0) -> (x*y=w418:dbl)
                "Velocity [deg/s]" <- w426
              }
              frame #1 {
                w494 = cluster{"output high":dbl, "output low":dbl} {"output high"=1.4, "output low"=-1.4}  # Output range
                n91 = local write "Velocity [deg/s] Chart"(w461) -> ()
                n92 = local write "Position End [deg]"(w459) -> ()
                n93 = local write "Position End [deg] Chart"(w459) -> ()
                n94 = First Call?() -> (First Call?: T/F=w484:bool)
                n95 = Or(x=w484, y=w483) -> (x .or. y?=w482:bool)
                n96 = Index Array(array=w464, index=w465) -> (element=w462:dbl)
                n97 = feedback #1() -> (w474:cluster{"time (s)":dbl, "setpoint":dbl}[])  [unwired: 1 in]
                n98 = case shown="True" w482 {
                  tunnel: [w501 w508] -> w473
                  tunnel: w474 -> [w501 _]
                  tunnel: w465 -> [w500 w504]
                  tunnel: w464 -> [_ w507]
                  tunnel: [w500 w503] -> w469
                  tunnel: w466 -> [_ w502]
                  frame False {
                  }
                  frame True {
                    # "Ramp time (s)"
                    # "Final Position"
                    n99 = Index Array(array=w507, index=w504) -> (element=w506:dbl)
                    n100 = call "Ramp_Trajectory_v2.vi"("Initial Time (s)"=0.0, "Period (s)"=0.01, "Ramp Duration (s)"=2.0, "Final Position (deg)"=w506, "Initial Position (deg)"=w502) -> ("Profile 2"=w508:cluster{"time (s)":dbl, "setpoint":dbl}[])  [unwired: 6 in]
                    n101 = Increment(x=w504) -> (x+1=w503:dbl)
                  }
                }
                n102 = feedback-in #1(w473) -> ()
                n103 = Greater Or Equal?(x=w462, y=185.0) -> (x >= y?=w468:bool)
                n104 = Unbundle By Name(T11 {"Gains"={"K(e)"=0.0, "Kp"=0.30000001192092896, "Ki"=0.10000000149011612, "Kd"=0.006000000052154064}, "Non-linear gain"={"Non-linear gain P"=enum."off", "Non-linear gain I"=enum."off", "Non-linear gain D"=enum."off"}, "D-Part variable"=enum."process variable", "Velocity estimate dy/dt"=enum."external", "Anti reset windup"=TRUE, "I-Part error band"=inf, "Output range"={"output high"=0.0, "output low"=0.0}} ("PID Settings")) -> ("Gains"=w493:T12, "Non-linear gain"=w492:T13, "D-Part variable"=w491:T15, "Velocity estimate dy/dt"=w490:T16, "Anti reset windup"=w489:bool, "I-Part error band"=w488:dbl)
                n105 = case shown="True" w468 {
                  tunnel: [FALSE TRUE] -> w467
                  frame False {
                  }
                  frame True {
                    n106 = local write "move"(FALSE) -> ()
                  }
                }
                n107 = call <vilib>:"PID Setpoint Profile.vi"("reinitialize? (F)"=w482, "dt (s)"=w485, "setpoint profile"=w473) -> ("profile complete?"=w472:bool, "setpoint"=w475:dbl)  [unwired: 3 in, 2 out]
                "Profile Complete?" <- w472
                n108 = call "ENPID.vi"(0:w475, 1:w481, 3:w490, 4:w486, 5:w485, 6:w493, "Reset?"=w489, "y"=w491, 10:w488, "dy/dt"=w492, 12:w494) -> (14:w471)  [unwired: 6 in, 2 out]
                n109 = case shown="True" w472 {
                  tunnel: [w498 0.0] -> w470
                  tunnel: w471 -> [w498 _]
                  frame False {
                  }
                  frame True {
                  }
                }
              }
              frame #2 {
                n110 = call "TF_MotorCurrentOutput.vi"("Motor Current Setpoint [A]"=w521) -> ("Motor Current Setpoint [V]"=w520:dbl)
                n111 = flat-sequence "Safety" {
                  tunnel: w520 -> [w537]
                  tunnel: [w522] -> w519
                  tunnel: w512 -> [w534]
                  frame #0 {
                    w527 = 0.0  # [V]
                    w523 = 0.0  # [V]
                    w535 = -175.0  # [deg]
                    w536 = 175.0  # [deg]
                    w529 = -1.0  # [V]
                    w533 = 1.0  # [V]
                    n112 = In Range and Coerce(upper limit=w533, x=w537, lower limit=w529) -> (coerced(x)=w530:dbl)  [unwired: 1 out]
                    n113 = Less Or Equal?(x=w534, y=w536) -> (x <= y?=w524:bool)
                    n114 = Greater Or Equal?(x=w534, y=w535) -> (x >= y?=w528:bool)
                    n115 = And(x=w524, y=w528) -> (x .and. y?=w525:bool)
                    n116 = Select(t=w533, s=w524, f=w523) -> (s? t:f=w531:dbl)
                    n117 = Select(t=w529, s=w528, f=w527) -> (s? t:f=w526:dbl)
                    n118 = In Range and Coerce(upper limit=w531, x=w530, lower limit=w526) -> (coerced(x)=w532:dbl)  [unwired: 1 out]
                    n119 = Select "Within Position Range?"(t=w530, s=w525, f=w532) -> (s? t:f=w522:dbl)
                  }
                }
              }
              frame #3 {
                # "Motor Current Setpoint"
                n120 = case shown="True" w541 {
                  tunnel: [TypeDef_Actions."Move" ("Actions") TypeDef_Actions."Wait" ("Actions")] -> w540
                  frame False {
                  }
                  frame True {
                  }
                }
                n121 = Build Array(w548) -> (w547:dbl[])
                n122 = call <vilib>:"Write.vi"("Values"=w547, "AO Ref In"=w545) -> ("AO Ref Out"=w546:T19)  [unwired: 7 in, 1 out]
              }
            }
          }
          frame "Wait" {
            n123 = Equal?(x=3000, y=w568) -> (x = y?=w576:bool)
            n124 = local write "Boolean: Apply Current"(FALSE) -> ()
            n125 = Select(t=0, s=w576, f=w568) -> (s? t:f=w574:i32)
            n126 = call <vilib>:"Read.vi"("Encoder Ref In"=w553) -> ("Counter Value"=w554:i32, "Encoder Ref Out"=w551:T27)  [unwired: 6 in, 3 out]
            n127 = Increment(x=w574) -> (x+1=w566:i32)
            n128 = case shown="False" w576 {
              tunnel: [TypeDef_Actions."Wait" ("Actions") TypeDef_Actions."Apply Current" ("Actions")] -> w579
              frame False {
              }
              frame True {
              }
            }
            n129 = Divide(x=w554, y=720000.0) -> (x/y=w556:dbl)
            n130 = Multiply(x=w556, y=360.0) -> (x*y=w552:dbl)
            n131 = Build Array(0.0) -> (w582:dbl[])
            n132 = local write "Boolean: Move"(FALSE) -> ()
            n133 = call <vilib>:"Write.vi"("Values"=w582, "AO Ref In"=w578) -> ("AO Ref Out"=w577:T19)  [unwired: 7 in, 1 out]
            n134 = local write "Position End [deg]"(w552) -> ()
            n135 = local write "Position End [deg] Chart"(w552) -> ()
            n136 = call <vilib>:"Read.vi"("Encoder Ref In"=w562) -> ("Counter Value"=w561:i32, "Encoder Ref Out"=w563:T27)  [unwired: 6 in, 3 out]
            n137 = call "TF_Encoder2Position.vi"("Counter Value"=w561, "Offset"=0.0) -> ("Position [deg]"=w559:dbl)  [unwired: 3 in]
          }
          frame "Apply Current" {
            n138 = flat-sequence {
              tunnel: w617 -> [w687]
              tunnel: w616 -> [w682]
              tunnel: [w674] -> w646
              tunnel: [w679] -> w645
              tunnel: w614 -> [w679]
              tunnel: w612 -> [w676]
              tunnel: [w677] -> w644
              tunnel: w610 -> [w673]
              tunnel: [w674] -> w643
              tunnel: [w673] -> w642
              tunnel: [w672] -> w641
              tunnel: w609 -> [w671]
              tunnel: [w671] -> w640
              tunnel: [w670] -> w639
              tunnel: w608 -> [w670]
              tunnel: [w669] -> w638
              tunnel: [w668] -> w637
              tunnel: w598 -> [w663]
              tunnel: [w662] -> w597
              tunnel: w596 -> [w661]
              tunnel: w591 -> [w653]
              tunnel: [w652] -> w587
              tunnel: [w651] -> w586
              tunnel: w646 -> [w703]
              tunnel: w645 -> [w714]
              tunnel: w644 -> [w717]
              tunnel: w643 -> [w715]
              tunnel: w642 -> [_]
              tunnel: w641 -> [w708]
              tunnel: [w701] -> w636
              tunnel: [w709] -> w635
              tunnel: [w716] -> w634
              tunnel: [w703] -> w633
              tunnel: [w709] -> w632
              tunnel: w640 -> [w713]
              tunnel: [w713] -> w631
              tunnel: [w712] -> w630
              tunnel: w639 -> [w712]
              tunnel: w638 -> [w711]
              tunnel: [w711] -> w629
              tunnel: [w710] -> w628
              tunnel: w637 -> [w710]
              tunnel: [w703] -> w627
              tunnel: w595 -> [w702]
              tunnel: [w699] -> w594
              tunnel: [w698] -> w588
              tunnel: w587 -> [w698]
              tunnel: w586 -> [w697]
              tunnel: w636 -> [w748]
              tunnel: [w748] -> w626
              tunnel: w635 -> [w753]
              tunnel: [w753] -> w625
              tunnel: w634 -> [w758]
              tunnel: [w758] -> w624
              tunnel: w633 -> [w747]
              tunnel: [w747] -> w623
              tunnel: w632 -> [w752]
              tunnel: [w750] -> w622
              tunnel: w631 -> [w757]
              tunnel: [w757] -> w621
              tunnel: w630 -> [w756]
              tunnel: [w756] -> w620
              tunnel: w629 -> [w755]
              tunnel: [w755] -> w619
              tunnel: w628 -> [w754]
              tunnel: [w754] -> w618
              tunnel: w627 -> [w749]
              tunnel: w594 -> [w746]
              tunnel: [w745] -> w593
              tunnel: [w744] -> w589
              tunnel: w588 -> [w744]
              tunnel: [w785] -> w611
              tunnel: [w786] -> w613
              tunnel: [w787] -> w615
              tunnel: [w777] -> w603
              tunnel: w626 -> [w777]
              tunnel: w625 -> [w787]
              tunnel: w624 -> [w786]
              tunnel: w623 -> [w785]
              tunnel: w622 -> [w783]
              tunnel: w621 -> [w782]
              tunnel: [w781] -> w606
              tunnel: [w780] -> w607
              tunnel: w620 -> [w780]
              tunnel: w619 -> [w779]
              tunnel: [w779] -> w605
              tunnel: w618 -> [w778]
              tunnel: [w778] -> w604
              tunnel: w593 -> [w776]
              tunnel: [w776] -> w592
              tunnel: [w775] -> w590
              tunnel: w589 -> [w775]
              frame #0 {
                n139 = call <vilib>:"Read.vi"("AI Ref In"=w687) -> ("Values"=w685:dbl[], "AI Ref Out"=w668:T29)  [unwired: 8 in, 1 out]
                n140 = Equal?(x=1, y=w676) -> (x = y?=w672:bool)
                n141 = flat-sequence {
                  tunnel: w650 -> [w694]
                  tunnel: [w690] -> w658
                  tunnel: w659 -> [w688]
                  frame #0 {
                    n142 = Reciprocal(x=w688) -> (1/x=w693:dbl)
                    n143 = call <vilib>:"Butterworth Filter PtByPt.vi"("order"=1, "filter type"=Filter_Passband_Type."Lowpass", "low cutoff freq: fl"=20.0, "sampling freq: fs"=w693, "x"=w694) -> ("Filtered x"=w690:dbl)  [unwired: 4 in, 1 out]
                  }
                }
                n144 = call <vilib>:"Read.vi"("Encoder Ref In"=w682) -> ("Counter Value"=w681:i32, "Encoder Ref Out"=w669:T27)  [unwired: 6 in, 3 out]
                n145 = call <vilib>:"Read.vi"("AI Ref In"=w663) -> ("Values"=w665:dbl[], "AI Ref Out"=w662:T29)  [unwired: 8 in, 1 out]
                n146 = Index Array(array=w685, index=0) -> (element=w684:dbl)
                n147 = call <vilib>:"Read.vi"("Encoder Ref In"=w653) -> ("Counter Value"=w654:i32, "Encoder Ref Out"=w652:T27)  [unwired: 6 in, 3 out]
                n148 = Divide(x=w661, y=1000000) -> (x/y=w659:dbl)
                n149 = call "TF_Encoder2Position.vi"("Counter Value"=w681, "Offset"=0.0) -> ("Position [deg]"=w674:dbl)  [unwired: 3 in]
                "Position [deg]" <- w674
                "Position [deg] Chart" <- w674
                n150 = Select(t=0, s=w672, f=w676) -> (s? t:f=w677:i32)
                n151 = Index Array(array=w665, index=0) -> (element=w649:dbl)
                n152 = call "TF_MotorCurrentInput.vi"("Motor Current Monitor Value [V]"=w684) -> ("Current [A]"=→"Current [A]" →"Current [A] Chart":dbl)
                n153 = call "TF_Tacho2Velocity_MIKE3.vi"("Motor Velocity Tacho Value [V]"=w649) -> ("Motor Velocity Tacho [deg/s]"=w650:dbl)  [unwired: 4 in]
                n154 = local write "Velocity [deg/s]"(w658) -> ()
                n155 = Divide(x=w654, y=720000.0) -> (x/y=w656:dbl)
                n156 = Multiply(x=w656, y=360.0) -> (x*y=w651:dbl)
                "Boolean: Apply Current" <- TRUE
                "Boolean: Move" <- FALSE
                "Velocity [deg/s] Chart" <- w658
              }
              frame #1 {
                n157 = case shown="\"Positive\", Default" "Current Direction" {
                  tunnel: w715 -> [w724 w729]
                  tunnel: [w723 w730] -> w701
                  tunnel: [w720 w726] -> w707
                  tunnel: "Pos Difference \nThreshold [deg]" -> [w719 w725]
                  frame "Positive", Default {
                    n158 = local read "Initial Position [deg]"() -> (w722:dbl)
                    n159 = Subtract(x=w724, y=w722) -> (x-y=w721:dbl)
                    n160 = Absolute Value(x=w721) -> (abs(x)=w720:dbl)
                    n161 = Greater Or Equal?(x=w720, y=w719) -> (x >= y?=w723:bool)
                  }
                  frame "Negative" {
                    n162 = local read "Initial Position [deg]"() -> (w728:dbl)
                    n163 = Subtract(x=w729, y=w728) -> (x-y=w727:dbl)
                    n164 = Absolute Value(x=w727) -> (abs(x)=w726:dbl)
                    n165 = Greater Or Equal?(x=w726, y=w725) -> (x >= y?=w730:bool)
                  }
                }
                "Position Difference [deg]" <- w707
                n166 = Increment(x=w717) -> (x+1=w716:i32)
                n167 = Equal?(x=w702, y=1.0) -> (x = y?=w704:bool)
                n168 = local write "Position End [deg]"(w697) -> ()
                n169 = local write "Position End [deg] Chart"(w697) -> ()
                n170 = case shown="True" w708 {
                  tunnel: w714 -> [w734 w737]
                  tunnel: [w734 w736] -> w706
                  tunnel: "Current Direction" -> [_ w735]
                  frame False {
                  }
                  frame True {
                    n171 = case shown="\"Negative\"" w735 {
                      tunnel: w737 -> [w739 w742]
                      tunnel: [w738 w741] -> w736
                      frame "Positive", Default {
                        w740 = 0.0001  # Current increment [A]
                        n172 = Add(x=w740, y=w739) -> (x+y=w738:dbl)
                      }
                      frame "Negative" {
                        w743 = 0.0001  # Current increment [A]
                        n173 = Subtract(x=w742, y=w743) -> (x-y=w741:dbl)
                      }
                    }
                  }
                }
                "Current Setpoint [A]" <- w706
                n174 = case shown="True" w704 {
                  tunnel: w703 -> [_ w718]
                  frame False {
                  }
                  frame True {
                    "Initial Position [deg]" <- w718
                  }
                }
                n175 = case shown="True" w701 {
                  tunnel: [w731 0.0] -> w709
                  tunnel: w706 -> [w731 w732]
                  frame False {
                  }
                  frame True {
                    "Final Current Setpoint" <- w732
                  }
                }
                n176 = Select(t=0.0, s=w701, f=w702) -> (s? t:f=w699:dbl)
              }
              frame #2 {
                n177 = call "TF_MotorCurrentOutput.vi"("Motor Current Setpoint [A]"=w752) -> ("Motor Current Setpoint [V]"=w751:dbl)
                n178 = flat-sequence "Safety" {
                  tunnel: w751 -> [w774]
                  tunnel: [w759] -> w750
                  tunnel: w749 -> [w771]
                  frame #0 {
                    w764 = 0.0  # [V]
                    w760 = 0.0  # [V]
                    w772 = -175.0  # [deg]
                    w773 = 175.0  # [deg]
                    w766 = -1.0  # [V]
                    w770 = 1.0  # [V]
                    n179 = In Range and Coerce(upper limit=w770, x=w774, lower limit=w766) -> (coerced(x)=w767:dbl)  [unwired: 1 out]
                    n180 = Less Or Equal?(x=w771, y=w773) -> (x <= y?=w761:bool)
                    n181 = Greater Or Equal?(x=w771, y=w772) -> (x >= y?=w765:bool)
                    n182 = And(x=w761, y=w765) -> (x .and. y?=w762:bool)
                    n183 = Select(t=w770, s=w761, f=w760) -> (s? t:f=w768:dbl)
                    n184 = Select(t=w766, s=w765, f=w764) -> (s? t:f=w763:dbl)
                    n185 = In Range and Coerce(upper limit=w768, x=w767, lower limit=w763) -> (coerced(x)=w769:dbl)  [unwired: 1 out]
                    n186 = Select "Within Position Range?"(t=w767, s=w762, f=w769) -> (s? t:f=w759:dbl)
                  }
                }
                n187 = Increment(x=w746) -> (x+1=w745:dbl)
              }
              frame #3 {
                # "Motor Current Setpoint"
                n188 = Build Array(w783) -> (w784:dbl[])
                n189 = call <vilib>:"Write.vi"("Values"=w784, "AO Ref In"=w782) -> ("AO Ref Out"=w781:T19)  [unwired: 7 in, 1 out]
              }
            }
            n190 = case shown="False" w603 {
              tunnel: [TypeDef_Actions."Apply Current" ("Actions") TypeDef_Actions."Move" ("Actions")] -> w602
              frame False {
              }
              frame True {
              }
            }
          }
        }
        n191 = Or(x="stop", y=w300) -> (x .or. y?=w301:bool)
        n192 = case shown="True" "stop" {
          frame False {
          }
          frame True {
            n193 = local write "move"(FALSE) -> ()
          }
        }
        n194 = node-c288() -> ()  [unwired: 1 in, 1 out]
      }
      n195 = node-c288(w169) -> ()  [unwired: 1 out]
      n196 = node-c288(w187) -> ()  [unwired: 1 out]
    }
    frame #5 {
      # "Encoder End Effector Side"
      # "Tachometer"
      # "Motor Current Monitor"
      # "Motor Current Setpoint"
      # "Encoder"
      # "Reset"
      # "Close Everything"
      n197 = call <vilib>:"Stop.vi"("Encoder Ref In"=w795) -> ("Encoder Ref Out"=w796:T27)  [unwired: 9 in, 1 out]
      n198 = call <vilib>:"Close.vi"("AI Ref In"=w798) -> ()  [unwired: 10 in, 1 out]
      n199 = Build Array(0.0) -> (w801:dbl[])
      n200 = call <vilib>:"Close.vi"("AI Ref In"=w797) -> ()  [unwired: 10 in, 1 out]
      n201 = call <vilib>:"Close.vi"("Encoder Ref In"=w796) -> ()  [unwired: 10 in, 1 out]
      n202 = call <vilib>:"Stop.vi"("Encoder Ref In"=w799) -> ("Encoder Ref Out"=w804:T27)  [unwired: 9 in, 1 out]
      n203 = call <vilib>:"Close.vi"("AO Ref In"=w805) -> ()  [unwired: 10 in, 1 out]
      n204 = call <vilib>:"Write.vi"("Values"=w801, "AO Ref In"=w800) -> ("AO Ref Out"=w803:T19)  [unwired: 7 in, 1 out]
      n205 = call <vilib>:"Close.vi"("Encoder Ref In"=w804) -> ()  [unwired: 10 in, 1 out]
      n206 = call <vilib>:"Close.vi"("AO Ref In"=w803) -> ()  [unwired: 10 in, 1 out]
    }
  }
